vi "measure_digital_FPGA.vi"() -> ()   [LabVIEW 2016]
uses:
  <vilib>/rvi/Emulation/niFpgaGetClockAttributes.vi
  <vilib>/rvi/Emulation/niFpgaSctlEmulationGetInTimedLoop.vi
  <vilib>/rvi/Emulation/niFpgaEmulationReportErrorSimple.vi
  <vilib>/rvi/Emulation/niFpgaProcessEmulError.vi
  <vilib>/rvi/eio/common/nirviEmuTemplateMethod_errors.vi
  <vilib>/rvi/Emulation/niFpgaCriticalErrorInLSC.vi
  <vilib>/eio/EIONode/EIONode.xnode
panel:
  out "Waveform Chart":i16(graph)
  out "x*y":u32
  out "negative flag":bool
  out "positive flag":bool
  out "Boolean":bool
  out "Numeric":i16
  in  "Sampling Interval for  1MHz\nFrequency (us)":u32=1
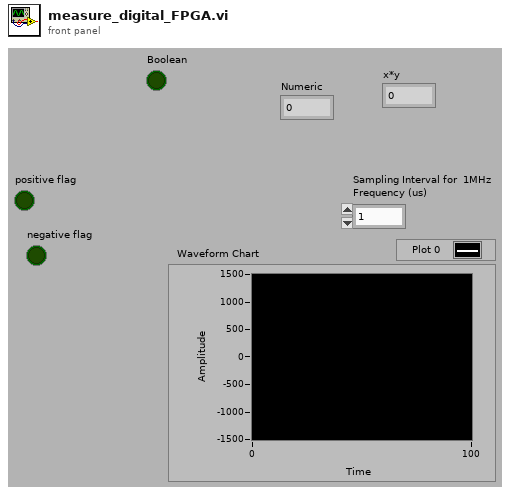
[diagram p1: front panel]
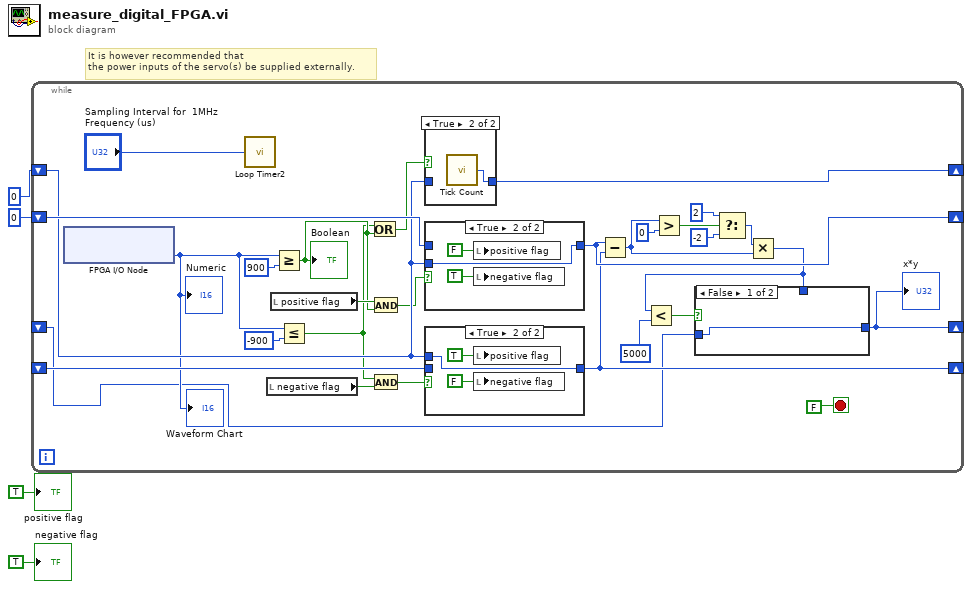
[diagram p0: block diagram]
diagram:
  # "It is however recommended that\nthe power inputs of the servo(s) be supplied externally."
  n1 = while {
    shift-right: [w33] -> _
    shift-left: u32 0 ("Tick Count(Ticks)") -> [w27]
    shift-right: [w24] -> _
    shift-left: u32 0 ("Tick Count(Ticks)") -> [w32]
    shift-right: [w23] -> _
    shift-left: _ -> [w25]
    shift-right: [w6] -> _
    shift-left: _ -> [w7]
    stop <- FALSE stop-if-true
    n2 = xnode "FPGA I/O Node"() -> ("AudioIn/Left"=w10:i16)  [unwired: 1 in, 1 out]
    "Numeric" <- w10
    "Waveform Chart" <- w10
    n3 = call "Loop Timer2"("Count(uSec)"="Sampling Interval for  1MHz\nFrequency (us)") -> ()  [unwired: 1 out]
    n4 = local read "negative flag"() -> (w12:bool)
    n5 = local read "positive flag"() -> (w15:bool)
    n6 = Greater Or Equal?(x=w10, y=i16 900) -> (x >= y?=w14:bool)
    "Boolean" <- w14
    n7 = Less Or Equal?(x=w10, y=i16 -900) -> (x <= y?=w11:bool)
    n8 = Or(x=w11, y=w14) -> (x .or. y?=w26:bool)
    n9 = And(x=w15, y=w14) -> (x .and. y?=w16:bool)
    n10 = And(x=w11, y=w12) -> (x .and. y?=w13:bool)
    n11 = case shown="True" w26 {
      tunnel: [w44 w45] -> w33
      tunnel: w27 -> [w44 _]
      frame False {
      }
      frame True {
        n12 = call "Tick Count"() -> ("Tick Count(uSec)"=w45:u32)
      }
    }
    n13 = case shown="True" w16 {
      tunnel: w32 -> [w40 _]
      tunnel: [w40 w43] -> w24
      tunnel: w27 -> [_ w43]
      frame False {
      }
      frame True {
        n14 = local write "positive flag"(FALSE) -> ()
        n15 = local write "negative flag"(TRUE) -> ()
      }
    }
    n16 = case shown="True" w13 {
      tunnel: w27 -> [_ w39]
      tunnel: [w36 w39] -> w23
      tunnel: w25 -> [w36 _]
      frame False {
      }
      frame True {
        n17 = local write "positive flag"(TRUE) -> ()
        n18 = local write "negative flag"(FALSE ("negative flag")) -> ()
      }
    }
    n19 = Subtract(x=w24, y=w23) -> (x-y=w17:u32)
    n20 = Greater?(x=w17, y=i16 0) -> (0:w19:bool)
    n21 = Select(t=i16 2, s=w19, f=i16 -2) -> (s? t:f=w18:i16)
    n22 = Multiply(x=w18, y=w17) -> (x*y=w8:u32)
    n23 = Less?(x=w8, y=i16 5000) -> (x < y?=w9:bool)
    n24 = case shown="False" w9 {
      tunnel: w8 -> [_ w35]
      tunnel: [w34 w35] -> w6
      tunnel: w7 -> [w34 _]
      frame False {
      }
      frame True {
      }
    }
    "x*y" <- w6
  }
  "positive flag" <- TRUE
  "negative flag" <- TRUE
